vi "XYGraph_to_Javascript3.vi"(5 "Captions":string[](array[string]), 7 "XY Graph":cluster{dbl[], dbl[]}[](array[cluster]), 8 "prename":string, 10 "file path (use dialog)":path) -> (0 "web page write":errorcluster)   [LabVIEW 2013]
doc: "Saves the xy graph to a javascript file usable by mjs_plot.js."
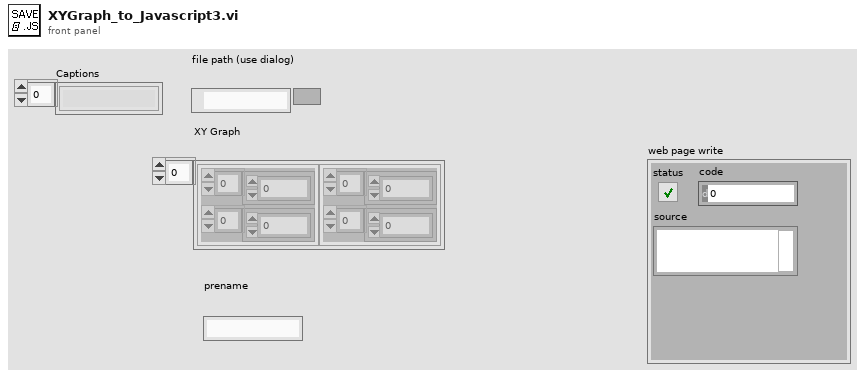
[diagram p1: front panel]
types:
  T1 = enum16{"open", "replace", "create", "open or create", "replace or create", "replace or create with confirmation"}
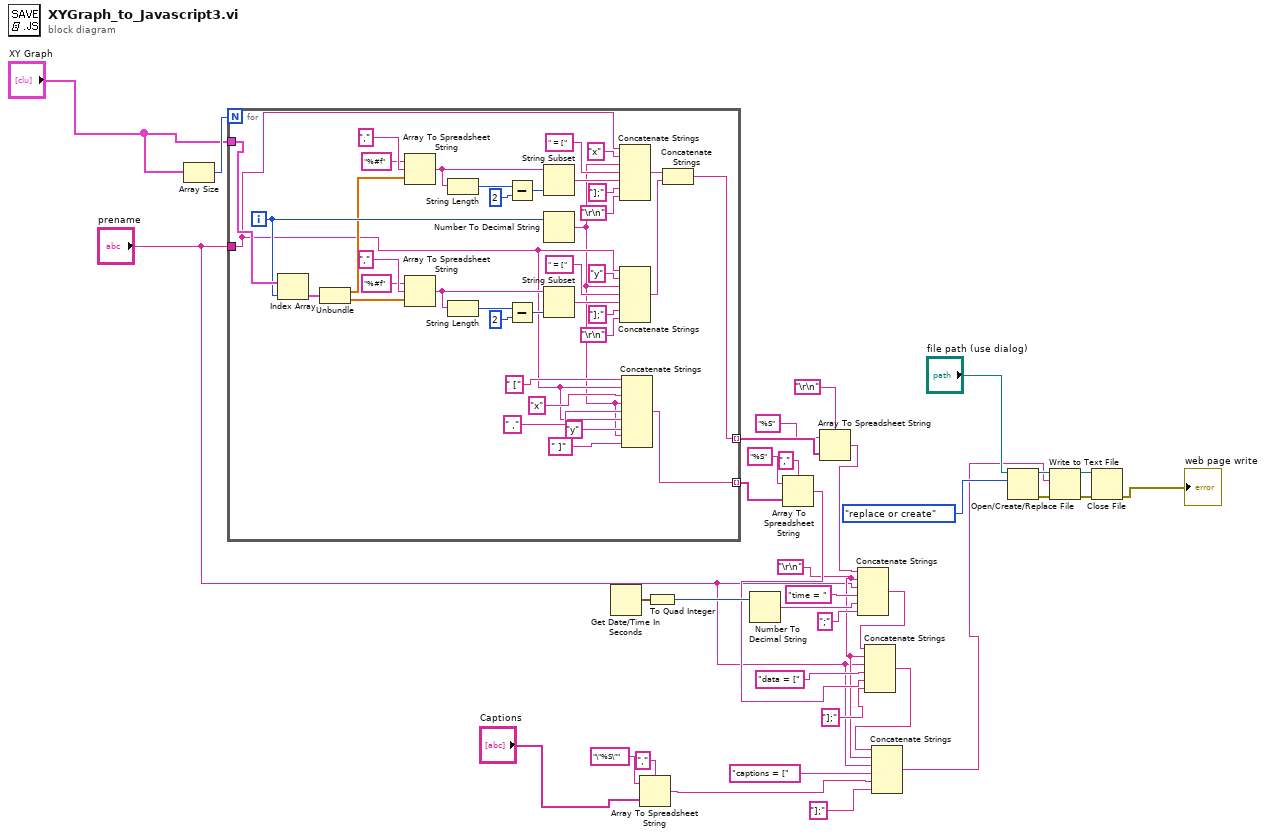
[diagram p0: block diagram]
diagram:
  w6 = "\r\n"
  n1 = Array Size(array="XY Graph") -> (size(s)=w35:i32)
  n2 = for {
    N: w35 -> [_]
    tunnel: "XY Graph" -> [w73]
    tunnel: [w47] -> w34 mode=indexing
    tunnel: "prename" -> [w39]
    tunnel: [w43] -> w17 mode=indexing
    i -> [w71]
    n3 = Index Array(array=w73, index=w71) -> (element=w46:cluster{dbl[], dbl[]})
    n4 = Unbundle(w46) -> (w45:dbl[], w44:dbl[])
    n5 = Array To Spreadsheet String(delimiter (Tab)="," ("string"), array=w45, 3:"%#f" ("format string")) -> (spreadsheet string=w57:string)
    n6 = Array To Spreadsheet String(delimiter (Tab)="," ("string"), array=w44, 3:"%#f" ("format string")) -> (spreadsheet string=w48:string)
    n7 = String Length(string=w57) -> (length=w55:i32)
    n8 = String Length(string=w48) -> (length=w52:i32)
    n9 = Subtract(x=w55, y=2) -> (x-y=w54:i32)
    n10 = Subtract(x=w52, y=2) -> (x-y=w51:i32)
    n11 = String Subset(string=w57, length (rest)=w54) -> (substring=w56:string)  [unwired: 1 in]
    n12 = Number To Decimal String(number=w71) -> (decimal integer string=w37:string)  [unwired: 1 in]
    n13 = String Subset(string=w48, length (rest)=w51) -> (substring=w49:string)  [unwired: 1 in]
    n14 = Concatenate Strings(w39, "x", w37, " = [", w56, "];", "\r\n") -> (w59:string)
    n15 = Concatenate Strings(w39, "y", w37, " = [", w49, "];", "\r\n") -> (w58:string)
    n16 = Concatenate Strings(" [", w39, "x", w37, " ,", w39, "y", w37, " ]") -> (w43:string)
    n17 = Concatenate Strings(w59, w58) -> (w47:string)
  }
  n18 = Get Date/Time In Seconds() -> (seconds since 1Jan1904=w23:timestamp)
  n19 = Array To Spreadsheet String(delimiter (Tab)=",", array="Captions", 3:"\"%S\"" ("format string")) -> (spreadsheet string=w3:string)
  n20 = To Quad Integer(1:w23) -> (0:w22:i64)
  n21 = Number To Decimal String(number=w22) -> (decimal integer string=w20:string)  [unwired: 1 in]
  n22 = Array To Spreadsheet String(delimiter (Tab)=",", array=w17, 3:"%S" ("format string")) -> (spreadsheet string=w12:string)
  n23 = Array To Spreadsheet String(delimiter (Tab)="\r\n", array=w34, 3:"%S" ("format string")) -> (spreadsheet string=w18:string)
  n24 = Concatenate Strings(w18, w6, "prename", "time = " ("string"), w20, ";" ("string")) -> (w14:string)
  n25 = Concatenate Strings(w14, w6, "prename", "data = [", w12, "];" ("string")) -> (w7:string)
  n26 = Concatenate Strings(w7, w6, "prename", "captions = [", w3, "];" ("string")) -> (w1:string)
  n27 = Open/Create/Replace File(file path (use dialog)="file path (use dialog)", operation (0:open)=T1."replace or create") -> (refnum out=w28:refnum<file>, error out=w25:errorcluster)  [unwired: 4 in, 1 out]
  n28 = Write to Text File(file (use dialog)=w28, text=w1, error in=w25) -> (refnum out=w27:refnum<file>, error out=w26:errorcluster)  [unwired: 1 in, 1 out]
  n29 = Close File(refnum=w27, error in=w26) -> (error out=→"web page write":errorcluster)  [unwired: 1 out]
